vi "niRFUtil MASMT 1D Inverse FFT (DBL).vi"(0 "FFT {X}":cdb[](array[numeric]), 1 "shift?":bool, 11 "error in (no error)":errorcluster) -> (4 "X":dbl[](array[numeric]), 15 "error out":errorcluster)   [LabVIEW 2015, in "niRFUtil.lvlib"]
doc: "Computes the inverse fast Fourier transform (FFT) of the input sequence <B>X</B>."
uses:
  niRFUtil.lvlib
  Utilities/niRFMASMT_FFT.dll
panel:
  out "workspace":dbl[](array[numeric])
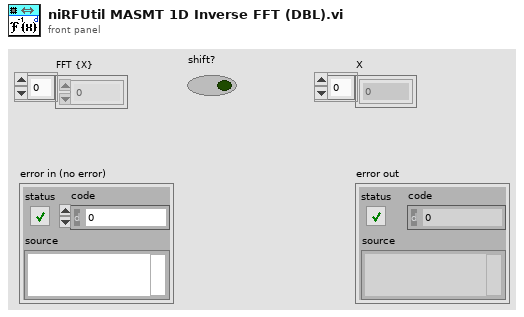
[diagram p1: front panel]
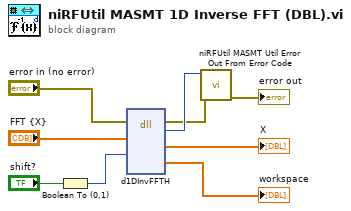
[diagram p0: block diagram]
diagram:
  n1 = Boolean To (0,1)(Boolean="shift?") -> (0, 1=w5:i16)
  n2 = dll-call lib="C:/Perforce/semoore-sales/Customers/NATI-3813/Noise Floor/LV Filters/ParallelComplexFilterRFUtil/niRFUtil/MASMT/Utilities/niRFMASMT_FFT.*" fn="d1DInvFFTH" ("lvanlys.dll:ReNIFFTH80")(error in="error in (no error)", "xH"="FFT {X}", "shift"=w5) -> (error out=w1:errorcluster, "return type"=w4:i32, "yH"=→"X":dbl[], "workspace"=→"workspace":dbl[])  [unwired: 8 in, 1 out]
  n3 = call "niRFUtil MASMT Util Error Out From Error Code.vi"("error in (no error)"=w1, "error code"=w4) -> ("error out"=→"error out":errorcluster)  [unwired: 9 in]
